vi "Shoot_Exec_SIM.vi"   [LabVIEW 2025]
uses:
  <vilib>/Rock Robotics/WPI/ThirdParty/JAS_Junk/TrajLib/Enum/DCMOTOR_TYPES_ENUM.ctl
  <vilib>/Rock Robotics/WPI/ThirdParty/JAS_Junk/TrajLib/BatterySim_CalculateLoadedBatteryVoltage.vi
  <vilib>/Rock Robotics/WPI/ThirdParty/JAS_Junk/TrajLib/Trajectory_Library.lvlib
types:
  T1 = typedef "Trajectory_Library.lvlib/DCMOTOR_TYPES_ENUM.ctl" = enum16{"CIM", "AndyMark 9015", "Andy Mark RS 775 125", "Bag", "BaneBots RS 550", "BaneBots RS 775", "Falcon 500", "Mini CIM", "NEO", "NEO 550", "Romi BuiltIn", "Vex 775 Pro", "Snow Blower AM 2235A", "Bosch Seat AM 3493", "Falcon 500 FOC", "Kraken X60", "Kraken X60 FOC", "NEO Vortex", "Minion", "Kraken X44", "Kraken X44 FOC"}
  T2 = typedef "Trajectory_Library.lvlib/LINEAR_SYSTEM_ID_FLYWHEEL_MODEL.ctl" = cluster{"DCMOTOR_TYPES":T1, "Num Motors":i32, "Gearing":dbl, "MOI kgm2":dbl}
  T3 = typedef "Trajectory_Library.lvlib/FLYWHEEL_SIM_SIMULATION_PARAMS.ctl" = cluster{"Vel Meas Std Dev Rad/Sec":dbl}
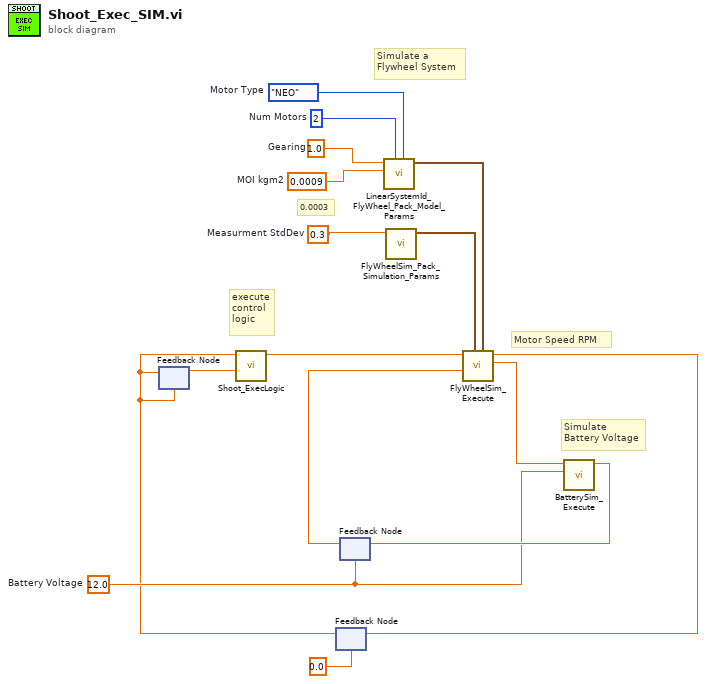
[diagram p0: block diagram]
diagram:
  w6 = 12.0  # Battery Voltage
  w10 = 0.3  # Measurment StdDev
  w13 = 1.0  # Gearing
  w14 = 0.0009  # MOI kgm2
  w15 = 2  # Num Motors
  w16 = DCMOTOR_TYPES_ENUM."NEO"  # Motor Type
  # "0.0003"
  # "execute\ncontrol\nlogic"
  # "Motor Speed RPM"
  # "Simulate\nBattery Voltage"
  # "Simulate a \nFlywheel System"
  n1 = feedback #1(0.0 ("Velocity_RPM")) -> (w1:dbl)
  n2 = feedback #2(w1) -> (w2:dbl)
  n3 = feedback-in #2(w1) -> ()
  n4 = call "Shoot_ExecLogic.vi"("Motor2Rpm"=w2, "Motor1Rpm"=w1) -> ("CO-ControlOutput"=w8:dbl)  [unwired: 9 in]
  n5 = feedback #3(w6) -> (w5:dbl)
  n6 = call <vilib>:"LinearSystemId_FlyWheel_Pack_Model_Params.vi"("DCMOTOR_TYPES"=w16, "Num Motors"=w15, "MOI kgm2"=w14, "Gearing"=w13) -> ("LinearSystem_ID_FlyWheel_Model"=w11:T2)  [unwired: 7 in]
  n7 = call <vilib>:"FlyWheelSim_Pack_Simulation_Params.vi"("Vel Meas StdDev Rad/Sec"=w10) -> ("FlyWheelSim_Simulation_Params"=w9:T3)  [unwired: 10 in]
  n8 = call <vilib>:"FlyWheelSim_Execute.vi"("FlyWheelSim_Model _Params"=w11, "FlyWheelSim_Simulation_Params"=w9, "Battery Volts"=w5, "Motor Dmd"=w8) -> ("Motor Current"=w12:dbl, "Velocity_RPM"=w4:dbl)  [unwired: 4 in, 2 out]
  n9 = feedback-in #1(w4) -> ()
  n10 = call <vilib>:"BatterySim_Execute.vi"("Nominal Battery Voltage"=w6, "Current"=w12) -> ("Voltage"=w7:dbl)  [unwired: 9 in]
  n11 = feedback-in #3(w7) -> ()
